vi "GetHiliteTextColor.vi"(8 "error in (no error)":errorcluster, 11 "Menu in":refnum<class "Menu.lvclass">) -> (0 "error out":errorcluster, 2 "HiliteTextColor":refnum<class "Color.lvclass">, 3 "Menu out":refnum<class "Menu.lvclass">)   [LabVIEW 2021, in "Menu.lvlib" / "Menu.lvclass"]
uses:
  Menu.lvclass
  Menu.lvclass/Menu.ctl
  Picture2D/src/Color/Color.lvclass
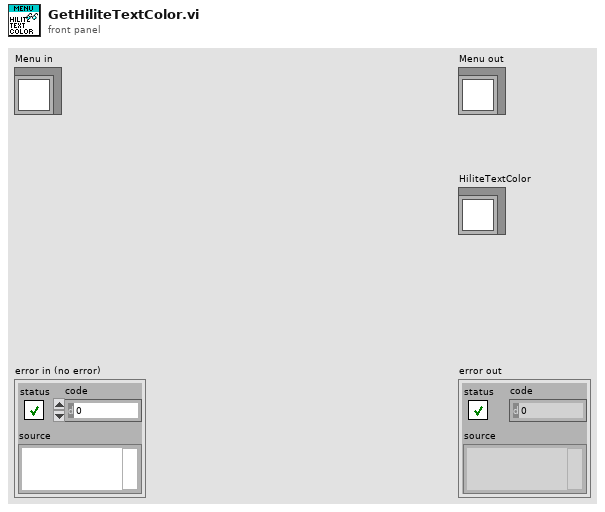
[diagram p1: front panel]
types:
  T1 = typedef "Menu.lvlib/Menu.lvclass/Data.ctl" = cluster{"MenuMap":map{string, T2}, "PictRef":refnum<vi>, "MenuSelectionEvent":refnum<user-event>, "TopMenuSpacing":i32, "MenuSpacing":i32, "CloseEvent":refnum<user-event>, "TR_ManageMenuRef":refnum<vi>, "MenuColors":T4, "RTMPath":path, "RTMVIReference":refnum<vi>, "RTMMenuReference":refnum<k9>, "CtlRef":refnum<vi>, "User-Specified Font":refnum<class "Font.lvclass">, "Desired Font":enum16{"User-specified Font", "Application Font", "System Font", "Dialog Font"}, "SubMenuIcon":T5, "SubMenuIconClosed":refnum<class "Picture2D.lvclass">, "SubMenuIconOpened":refnum<class "Picture2D.lvclass">}
  T2 = typedef "Menu.lvlib/Menu.lvclass/MenuItems.ctl" = cluster{"Item Name":string, "Short Cut":T3, "Checked":bool, "Enable":bool, "After item":string, "Item Tags":string[], "Item Names":string[], "Picture":refnum<class "Image.lvclass">, "Hilite Picture":refnum<class "Image.lvclass">, "Displayed":bool}
  T3 = typedef "LVMenuShortCut.ctl" = cluster{"Include Shift Key?":bool, "Include Ctrl Key?":bool, "Shortcut Key":string}
  T4 = typedef "Menu.lvlib/Menu.lvclass/MenuColors.ctl" = cluster{"Text":refnum<class "Color.lvclass">, "HiliteText":refnum<class "Color.lvclass">, "Background":refnum<class "Color.lvclass">, "BorderColor":refnum<class "Color.lvclass">, "Hilite":refnum<class "Color.lvclass">}
  T5 = typedef "Menu.lvlib/Menu.lvclass/SubMenuIcon.ctl" = enum16{"LabVIEW", "Windows", "Custom"}
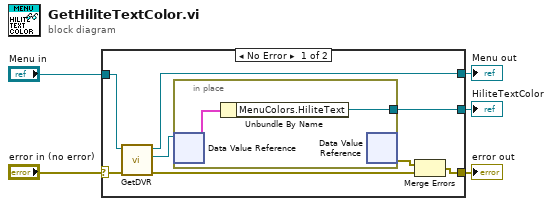
[diagram p0: block diagram]
diagram:
  n1 = case shown="No Error" "error in (no error)" {
    selector: "error in (no error)" -> [w13 w17]
    tunnel: [w8 w17] -> w4
    tunnel: [w11 w16] -> w2
    tunnel: "Menu in" -> [w10 w16]
    tunnel: [w6 _] -> w1
    frame No Error {
      n2 = call "GetDVR.vi"("error in (no error)"=w13, "Menu in"=w10) -> ("error out"=w12:errorcluster, "DVR"=w9:refnum<data-value>, "Menu out"=w11:refnum<class "Menu.lvclass">)  [unwired: 7 in]
      n3 = in-place {
        in-place-border: [w14] -> w6
        n4 = in-place-dvr #1(w9) -> (w15:T1)  [unwired: 1 out]
        n5 = Unbundle By Name(w15) -> ("MenuColors.HiliteText"=w14:refnum<class "Color.lvclass">)
        n6 = in-place-dvr #1() -> (w7:errorcluster)  [unwired: 1 in, 1 out]
      }
      n7 = Merge Errors(w7, w12) -> (w8:errorcluster)
    }
    frame Error {
    }
  }
  "error out" <- w4
  "Menu out" <- w2
  "HiliteTextColor" <- w1
